vi "MSEncoder Case-13-UpdRFChScale.vi"(8 "error in (no error)":errorcluster, 9 "ParamValIn":variant, 11 "MSEncoder in":refnum<class "MSEncoder.lvclass">) -> (0 "error out":errorcluster, 3 "MSEncoder out":refnum<class "MSEncoder.lvclass">)   [LabVIEW 2018, in "MSEncoder.lvclass"]
uses:
  MSEncoder.lvclass
  Ctl/MSEditorParam updRFScale.ctl
  MSEncoder.lvclass/MSEncoder.ctl
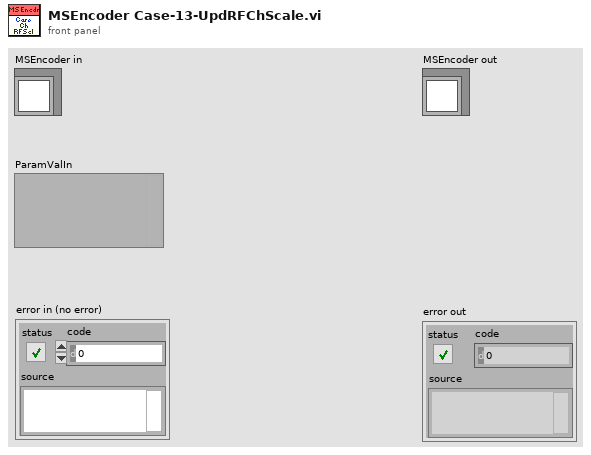
[diagram p1: front panel]
types:
  T1 = typedef "MSEditorParam updRFScale.ctl" = cluster{"ch1":dbl, "ch2":dbl, "ch3":dbl}
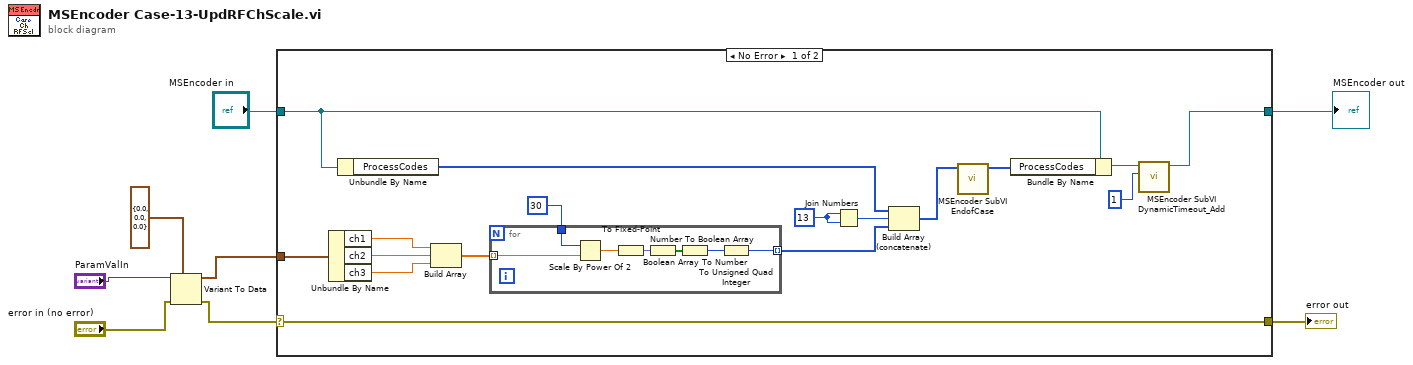
[diagram p0: block diagram]
diagram:
  n1 = Variant To Data(error in="error in (no error)", type=T1 {"ch1"=0.0, "ch2"=0.0, "ch3"=0.0} ("ParamValueType"), Variant="ParamValIn") -> (data=w3:T1, error out=w2:errorcluster)
  n2 = case shown="No Error" w2 {
    selector: w2 -> [w19 w34]
    tunnel: "MSEncoder in" -> [w24 w33]
    tunnel: [w19 w34] -> w8
    tunnel: [w16 w33] -> w7
    tunnel: w3 -> [w18 _]
    frame No Error {
      w22 = u32 13
      n3 = Unbundle By Name(w18) -> ("ch1"=w14:dbl, "ch2"=w13:dbl, "ch3"=w12:dbl)
      n4 = Unbundle By Name(w24) -> ("ProcessCodes"=w25:u64[])
      n5 = Build Array(w14, w13, w12) -> (w11:dbl[])
      n6 = for {
        tunnel: w11 -> [w28] mode=indexing
        tunnel: [w27] -> w9 mode=indexing
        tunnel: i16 30 ("n") -> [w26]
        n7 = Scale By Power Of 2(n=w26, x=w28) -> (x*2^n=w29:dbl)
        n8 = To Fixed-Point(number=w29) -> (fixed-point=w30:fxp<+,32,32>)  [unwired: 1 in]
        n9 = Number To Boolean Array(number=w30) -> (Boolean array=w31:bool[])
        n10 = Boolean Array To Number(Boolean array=w31) -> (number=w32:u32)
        n11 = To Unsigned Quad Integer(1:w32) -> (0:w27:u64)
      }
      n12 = Join Numbers(hi=w22, lo=w22) -> ((hi.lo)=w21:u64)
      n13 = Build Array (concatenate)(w25, w21, w9) -> (w20:u64[])
      n14 = call "MSEncoder SubVI EndofCase.vi"("Case codes"=w20) -> ("Case codes with end"=w23:u64[])  [unwired: 9 in, 1 out]
      n15 = Bundle By Name(cluster=w24, "ProcessCodes"=w23) -> (w17:refnum<class "MSEncoder.lvclass">)
      n16 = call "MSEncoder SubVI DynamicTimeout_Add.vi"("Timeout_ms"=1, "MSEncoder"=w17) -> ("MSEncoder"=w16:refnum<class "MSEncoder.lvclass">)  [unwired: 8 in, 1 out]
    }
    frame Error {
    }
  }
  "error out" <- w8
  "MSEncoder out" <- w7
